vi "Init WS Manager.vi"(8 "error in (no error)":errorcluster, 11 "WebSocket Manager in":refnum<class "WebSocket Manager.lvclass">) -> (0 "error out":errorcluster, 3 "WebSocket Manager out":refnum<class "WebSocket Manager.lvclass">)   [LabVIEW 2020, in "HTTP Server.lvlib" / "WebSocket Manager.lvclass"]
uses:
  WebSocket Manager.lvclass
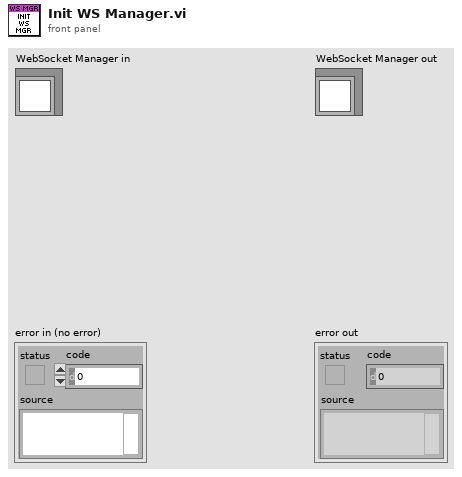
[diagram p1: front panel]
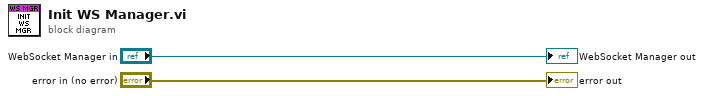
[diagram p0: block diagram]
diagram:
  "error out" <- "error in (no error)"
  "WebSocket Manager out" <- "WebSocket Manager in"
